vi "GET_DownloadFile_Async.vi"(4 "Prefered Stat Scale [MB]":T2=1000000 items=["Bytes"=1, "KB"=1000, "MB"=1000000, "GB"=1000000000], 6 "Timeout_ms (10000)":i32=10000, 7 "TargetFilePath":path, 8 "error in (no error)":errorcluster, 10 "URL":string, 11 "LabVIEWHTTPClient_NET in":refnum<class "HttpClient_NET.lvclass">) -> (0 "error out":errorcluster, 2 "DownloadTask Ref":T1, 3 "LabVIEWHTTPClient_NET out":refnum<class "HttpClient_NET.lvclass">)   [LabVIEW 2018, in "HttpClient_NET.lvlib" / "HttpClient_NET.lvclass"]
doc: "<b> </b> <b> </b>\nHttpClient_NET\nJustin Young - Viviota\nCopyright (c) 2021\nLicense: BSD"
uses:
  HttpClient_NET.lvclass
  Types/ScaledValue_ring.ctl
  HttpDownloadTask/Types/DownloadTask_ref.ctl
  HttpDownloadTask/HttpDownloadTask.lvclass
  Types/method_enum.ctl
  HttpClient_NET.lvclass/HttpClient_NET.ctl
  Accessors/Write RequestHeaderContentFirst.vi
  HttpClient_NET.lvlib
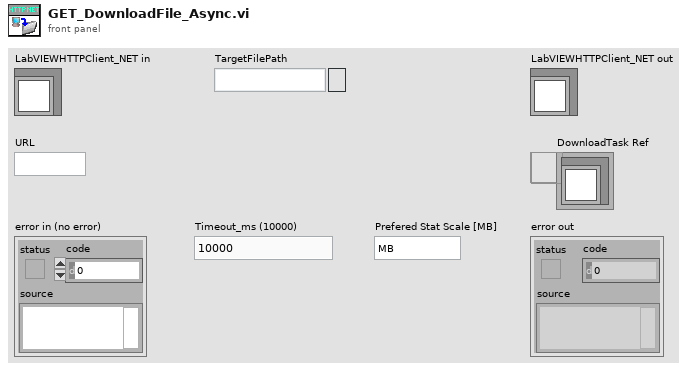
[diagram p1: front panel]
types:
  T1 = typedef "HttpClient_NET.lvlib/HttpDownloadTask.lvclass/DownloadTask_ref.ctl" = refnum<data-value>
  T2 = typedef "HttpClient_NET.lvlib/ScaledValue_ring.ctl" = u64
  T3 = typedef "HttpClient_NET.lvlib/method_enum.ctl" = enum16{"GET", "PUT", "POST", "DELETE", "HEAD", "TRACE", "SEND"}
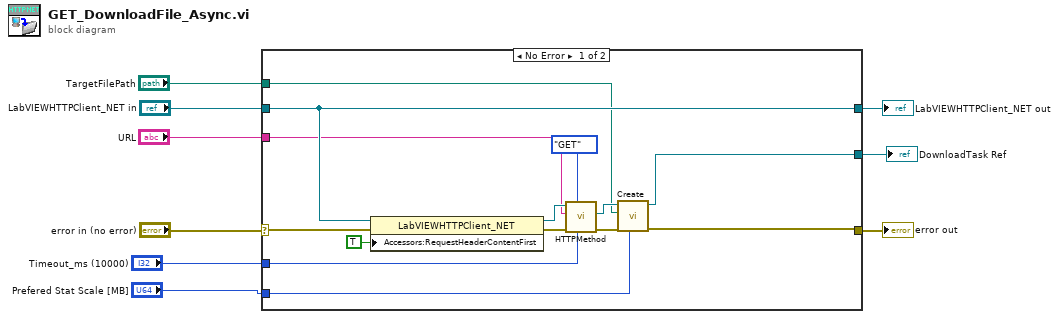
[diagram p0: block diagram]
diagram:
  n1 = case shown="No Error" "error in (no error)" {
    selector: "error in (no error)" -> [w18 w25]
    tunnel: [w14 w25] -> w8
    tunnel: [w17 w24] -> w6
    tunnel: "LabVIEWHTTPClient_NET in" -> [w17 w24]
    tunnel: "URL" -> [w16 _]
    tunnel: "Prefered Stat Scale [MB]" -> [w13 _]
    tunnel: "Timeout_ms (10000)" -> [w12 _]
    tunnel: "TargetFilePath" -> [w11 _]
    tunnel: [w10 _] -> w1
    frame No Error {
      n2 = property class="LabVIEWHTTPClient_NET"(reference=w17, error in=w18, "Accessors:RequestHeaderContentFirst"=TRUE ("RequestHeaderContentFirst")) -> (reference out=w21:refnum<class "HttpClient_NET.lvclass">, error out=w22:errorcluster)
      n3 = call "HTTPMethod.vi"("Timeout_ms (10000)"=w12, "Method"=method_enum."GET", "error in (no error)"=w22, "URL"=w16, "LabVIEWHTTPClient_NET in"=w21) -> ("error out"=w15:errorcluster, "HttpResponseMessage out"=w19:refnum<class "HttpResponseMessage.lvclass">)  [unwired: 4 in, 1 out]
      n4 = call "Create.vi"("Prefered Scale [MB]"=w13, "error in (no error)"=w15, "FilePath"=w11, "HttpResponseMessage"=w19) -> ("error out"=w14:errorcluster, "DownloadTask Ref"=w10:T1)  [unwired: 6 in]
    }
    frame Error {
    }
  }
  "error out" <- w8
  "LabVIEWHTTPClient_NET out" <- w6
  "DownloadTask Ref" <- w1
